vi "set_sample_parameters.vi"(8 "Error In":errorcluster) -> (0 "Error Out":errorcluster)   [LabVIEW 2019]
uses:
  sample_parameter_cluster_typedef.ctl
  set_sample_parameters_states_enum_typedef.ctl
panel:
  in  "Cancel":bool
  in  "Done":bool
  in  "Get c Parameter":bool
  in  "Samples":i32(listbox)
  in  "Sample Parameters":T1
  in  "Get Samples":bool
  in  "Data Directory":path
  # "Set Sample Parameters"
  # "1. Set the data directory and click \"Get Samples\"\n2. Select the sample to analyze from the list\n3. Click \"Get c Parameter\" and determine c\n4. Fill in the sample parameters\n5. Click done to save and close"
  # "Air"
  # "Glass"
  # "Ice"
  # "mm"
  # "mm"
  # "mm/px"
  # "px"
  # "px"
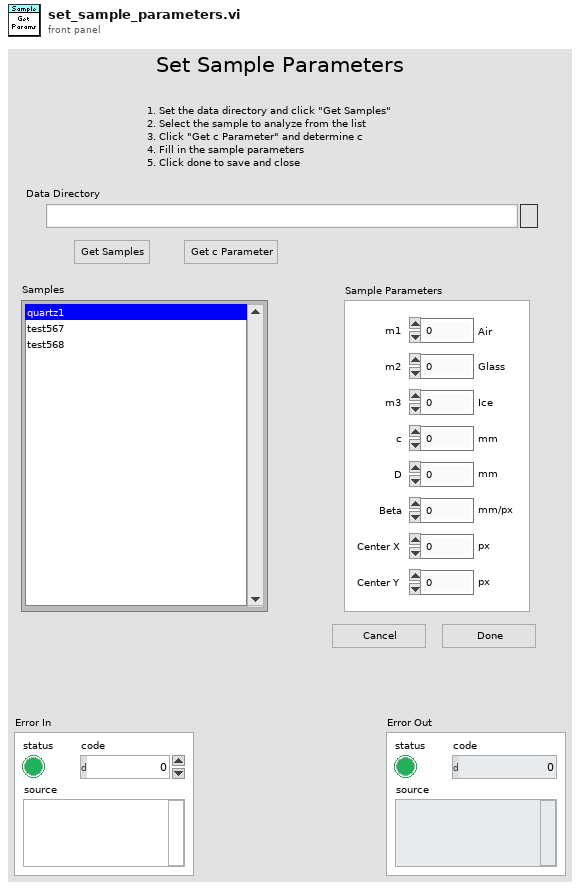
[diagram p1: front panel]
types:
  T1 = typedef "sample_parameter_cluster_typedef.ctl" = cluster{"m1":dbl, "m2":dbl, "m3":dbl, "c":dbl, "D":dbl, "Beta":dbl, "Center X":dbl, "Center Y":dbl}
  T2 = typedef "set_sample_parameters_states_enum_typedef.ctl" = enum16{"Shutdown", "Save", "Get c Parameter", "Get Samples", "Wait", "Initialize"}
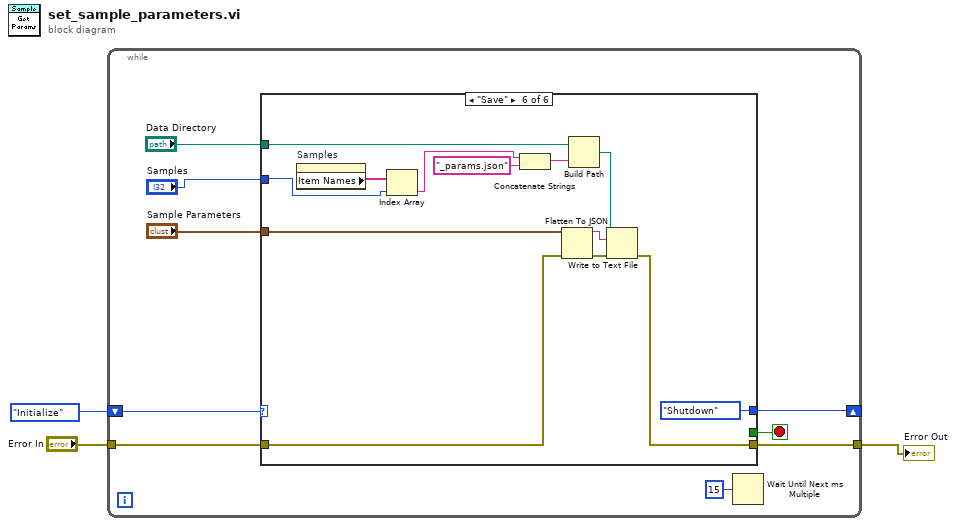
[diagram p0: block diagram]
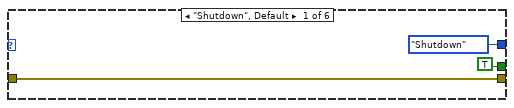
[diagram p2: hidden frame]
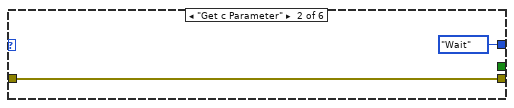
[diagram p3: hidden frame]
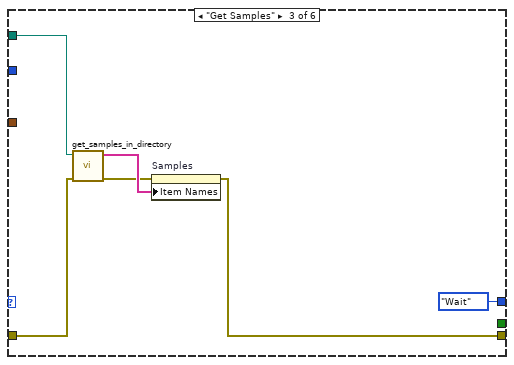
[diagram p4: hidden frame]
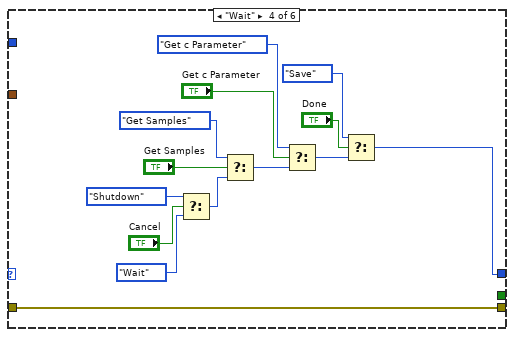
[diagram p5: hidden frame]
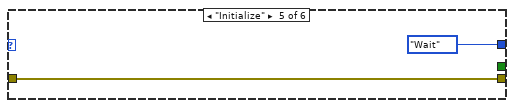
[diagram p6: hidden frame]
diagram:
  n1 = while {
    tunnel: "Error In" -> [w12]
    shift-right: [w10] -> _
    shift-left: set_sample_parameters_states_enum_typedef."Initialize" -> [w11]
    tunnel: [w8] -> w1
    stop <- w6 stop-if-true
    n2 = case shown="\"Save\"" w11 {
      tunnel: w12 -> [w15 w16 w22 w28 w38 w49]
      tunnel: [set_sample_parameters_states_enum_typedef."Shutdown" set_sample_parameters_states_enum_typedef."Wait" set_sample_parameters_states_enum_typedef."Wait" w29 set_sample_parameters_states_enum_typedef."Wait" set_sample_parameters_states_enum_typedef."Shutdown"] -> w10
      tunnel: [w15 w16 w19 w28 w38 w40] -> w8
      tunnel: "Data Directory" -> [_ _ w23 _ _ w46]
      tunnel: [TRUE _ _ _ _ _] -> w6
      tunnel: "Samples" -> [_ _ _ _ _ w42]
      tunnel: "Sample Parameters" -> [_ _ _ _ _ w50]
      frame "Shutdown", Default {
      }
      frame "Get c Parameter" {
      }
      frame "Get Samples" {
        n3 = call "get_samples_in_directory.vi"("Error In"=w22, "Data Directory"=w23) -> ("Error Out"=w20:errorcluster, "Samples"=w21:string[])  [unwired: 8 in]
        n4 = property on="Samples" class="LstBox (strict)"(error in=w20, "Item Names"=w21) -> (error out=w19:errorcluster)  [unwired: 1 in, 1 out]
      }
      frame "Wait" {
        n5 = Select(t=set_sample_parameters_states_enum_typedef."Shutdown", s="Cancel", f=set_sample_parameters_states_enum_typedef."Wait") -> (s? t:f=w26:T2)
        n6 = Select(t=set_sample_parameters_states_enum_typedef."Get Samples", s="Get Samples", f=w26) -> (s? t:f=w37:T2)
        n7 = Select(t=set_sample_parameters_states_enum_typedef."Get c Parameter", s="Get c Parameter", f=w37) -> (s? t:f=w36:T2)
        n8 = Select(t=set_sample_parameters_states_enum_typedef."Save", s="Done", f=w36) -> (s? t:f=w29:T2)
      }
      frame "Initialize" {
      }
      frame "Save" {
        n9 = property on="Samples" class="LstBox (strict)"() -> ("Item Names"=w51:string[])  [unwired: 2 in, 2 out]
        n10 = Index Array(array=w51, index=w42) -> (element=w43:string)
        n11 = Concatenate Strings(w43, "_params.json" ("string")) -> (w45:string)
        n12 = Flatten To JSON(anything=w50, error in (no error)=w49) -> (JSON string=w47:string, 11:w48:errorcluster)  [unwired: 1 in]
        n13 = Build Path(base path=w46, name or relative path=w45) -> (appended path=w41:path)
        n14 = Write to Text File(file (use dialog)=w41, text=w47, error in=w48) -> (error out=w40:errorcluster)  [unwired: 1 in, 2 out]
      }
    }
    n15 = Wait Until Next ms Multiple(millisecond multiple=u32 15) -> ()  [unwired: 1 out]
  }
  "Error Out" <- w1
